vi "Acquire Image.vi"(8 "error in (no error)":errorcluster, 11 "ImageHandler in":refnum<class "ImageHandler.lvclass">) -> (0 "error out":errorcluster, 3 "ImageHandler out":refnum<class "ImageHandler.lvclass">)   [LabVIEW 2022 SP3, in "ImageHandler.lvlib" / "ImageHandler.lvclass"]
uses:
  ImageHandler.lvclass
  BonTechDetector/Controls/Acquisition Commands.ctl
  ImageHandler.lvclass/ImageHandler.ctl
  BonTechDetector/BonTechDetector.lvlib
  <vilib>/ActorFramework/Actor/Actor.lvclass
  ImageHandler - Controller -- Interface/ImageHandler - Controller -- Interface Messages/Log Message Msg/Log Message Msg.lvclass
  C:/Program Files/National Instruments/LabVIEW 2022/vi.lib/ActorFramework/Actor/Actor.lvclass
  E:/GitHub/image-harvest/ImageHandler/ImageHandler/ImageHandler.lvclass
panel:
  out "function return":i32
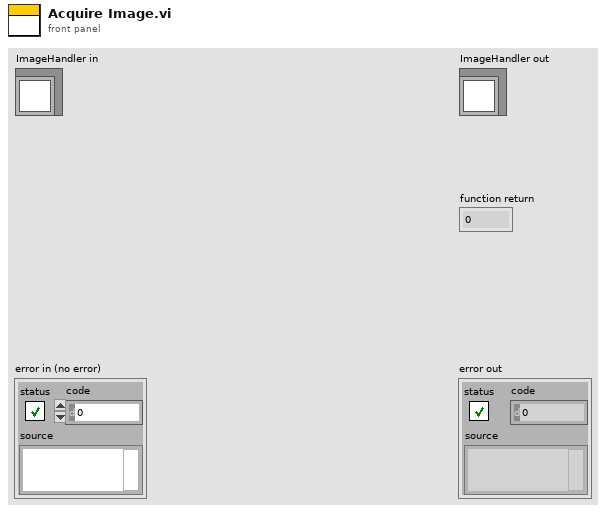
[diagram p1: front panel]
types:
  T1 = typedef "BonTechDetector.lvlib/Acquisition Commands.ctl" = u32
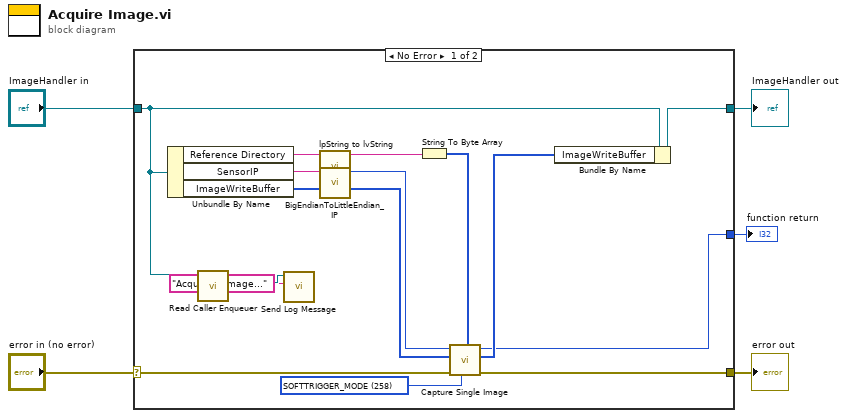
[diagram p0: block diagram]
diagram:
  n1 = case shown="No Error" "error in (no error)" {
    selector: "error in (no error)" -> [w20 w22]
    tunnel: [w19 w22] -> w4
    tunnel: [w12 w21] -> w2
    tunnel: "ImageHandler in" -> [w8 w21]
    tunnel: [w10 _] -> w1
    frame No Error {
      w16 = T1 258 items=["ACQ_INIT"=0, "DARK_MODE"=1, "BRIGHT_MODE"=2, "SOFTTRIGGER_MODE"=258, "SOFTTRIGGER_INSTANT_MODE"=259] ("nMode")
      n2 = Unbundle By Name(w8) -> ("Reference Directory"=w15:string, "SensorIP"=w18:string, "ImageWriteBuffer"=w9:u16[])
      n3 = call <vilib>:"Read Caller Enqueuer.vi"("Actor"=w8) -> ("Caller Enqueuer"=w7:refnum<class "Message Enqueuer.lvclass">)  [unwired: 10 in]
      n4 = call "Send Log Message.vi"("Log Message"="Acquiring Image...", "Message Enqueuer"=w7) -> ()  [unwired: 8 in, 2 out]
      n5 = call "lpString to lvString.vi"("LPTSTR String"=w15) -> ("LVString"=w13:string)  [unwired: 10 in]
      n6 = call "BigEndianToLittleEndian_IP.vi"("IP String"=w18) -> ("IP Network Order"=w17:u32)  [unwired: 10 in]
      n7 = String To Byte Array(string=w13) -> (unsigned byte array=w14:u8[])
      n8 = call "Capture Single Image.vi"("calRefPath"=w14, "nMode"=w16, "error in (no error)"=w20, "pImage"=w9, "nSensorIP"=w17) -> ("error out"=w19:errorcluster, "pImage out"=w11:u16[], "function return"=w10:i32)  [unwired: 4 in]
      n9 = Bundle By Name(cluster=w8, "ImageWriteBuffer"=w11) -> (w12:refnum<class "ImageHandler.lvclass">)
    }
    frame Error {
    }
  }
  "error out" <- w4
  "ImageHandler out" <- w2
  "function return" <- w1
